vi "insertNode.vi"(8 "error in (no error)":errorcluster, 10 "node ref in":refnum<data-value>, 11 "InconsistentList in":refnum<class "NI_Robotics_InconsistentList.lvclass">) -> (0 "error out":errorcluster, 3 "InconsistentList out":refnum<class "NI_Robotics_InconsistentList.lvclass">)   [LabVIEW 2017, in "NI_Robotics_InconsistentList.lvclass"]
uses:
  <vilib>/robotics/Navigation/shared/InconsistentList/NI_Robotics_InconsistentList.lvclass
  <vilib>/robotics/Navigation/shared/MapNode/AbstractDstarNode/NI_Robotics_AbstractDstarNode.lvclass
  <vilib>/robotics/Navigation/shared/InconsistentList/NI_Robotics_InconsistentList.lvclass/NI_Robotics_InconsistentList.ctl
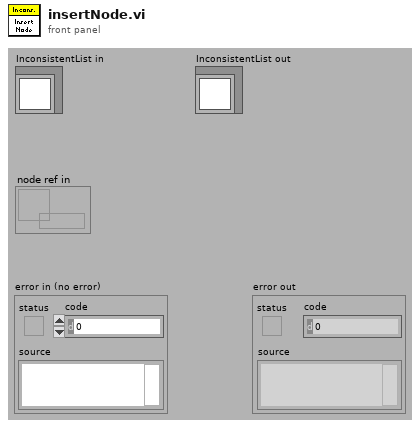
[diagram p1: front panel]
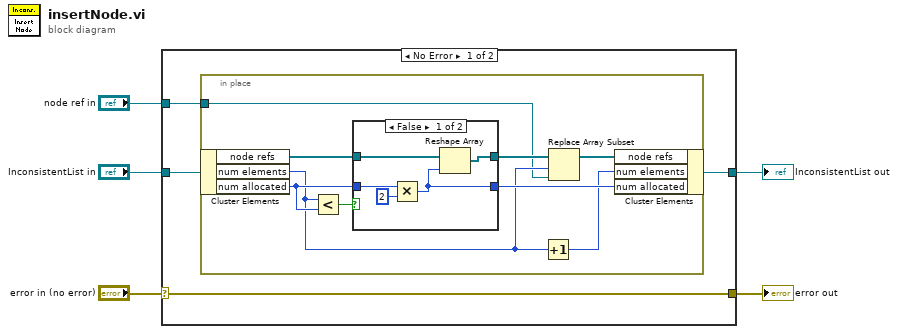
[diagram p0: block diagram]
diagram:
  n1 = case shown="No Error" "error in (no error)" {
    selector: "error in (no error)" -> [w7 w26]
    tunnel: "InconsistentList in" -> [w9 w27]
    tunnel: [w8 w27] -> w4
    tunnel: "node ref in" -> [w6 _]
    tunnel: [w7 w26] -> w1
    frame No Error {
      n2 = in-place {
        in-place-border: w6 -> [w10]
        n3 = in-place-cluster #1(w9) -> ("node refs"=w15:refnum<data-value>[], "num elements"=w11:i32, "num allocated"=w17:i32)
        n4 = Less?(x=w11, y=w17) -> (x < y?=w18:bool)
        n5 = case shown="False" w18 {
          tunnel: w17 -> [w21 w25]
          tunnel: [w19 w25] -> w16
          tunnel: w15 -> [w23 w24]
          tunnel: [w22 w24] -> w12
          frame False {
            n6 = Multiply(x=w21, y=2) -> (x*y=w19:i32)
            n7 = Reshape Array(w23, w19) -> (w22:refnum<data-value>[])
          }
          frame True {
          }
        }
        n8 = Increment(x=w11) -> (x+1=w14:i32)
        n9 = Replace Array Subset(array=w12, new element=w10, index=w11) -> (w13:refnum<data-value>[])
        n10 = in-place-cluster #1("node refs"=w13, "num elements"=w14, "num allocated"=w16) -> (w8:refnum<class "NI_Robotics_InconsistentList.lvclass">)
      }
    }
    frame Error {
    }
  }
  "InconsistentList out" <- w4
  "error out" <- w1
